vi "get_firmware_version_number.vi"(8 "error in (no error)":errorcluster, 11 "VISA resource name":refnum<visa-resource-name>) -> (0 "error out":errorcluster, 2 "Firmware version number":sgl, 3 "VISA resource name out":refnum<visa-resource-name>)   [LabVIEW 2018, in "Inficon IC6.lvlib"]
doc: "Query the firmware version number."
uses:
  <instrlib>/Inficon IC6/Inficon IC6.lvlib
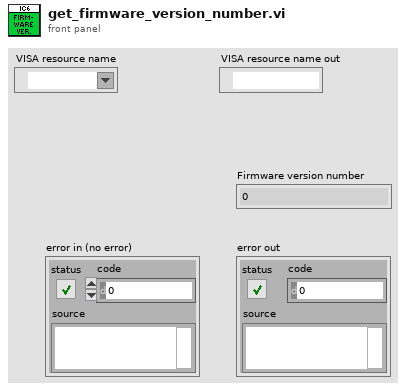
[diagram p1: front panel]
types:
  T1 = enum16{"Source", "General", "Input name", "Process name", "Logic", "Material", "Material name", "Output name", "Process", "Sensor", "Output type", "User message", "Layer", ""}
  T2 = enum16{"Hello", "Query", "Remote action", "Status", "Update"}
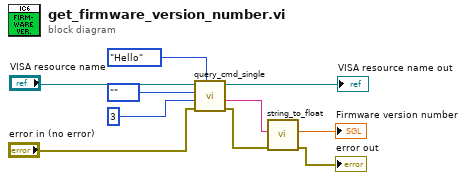
[diagram p0: block diagram]
diagram:
  n1 = call <instrlib>:"query_cmd_single.vi"("Command group"=T2."Hello", "error in (no error)"="error in (no error)", "Command ID"=u8 3, "Command subgroup"=T1."", "VISA resource name"="VISA resource name") -> ("error out"=w4:errorcluster, "formatted response"=w5:string, "VISA resource name out"=→"VISA resource name out":refnum<visa-resource-name>)  [unwired: 2 in, 2 out]
  n2 = call <instrlib>:"string_to_float.vi"("error in (no error)"=w4, "Float (string)"=w5) -> ("error out"=→"error out":errorcluster, "Float (sgl)"=→"Firmware version number":sgl)  [unwired: 8 in]
